vi "Connect.vi"(11 "Device Serial Number":string) -> (1 "Handle":u64, 3 "FT_Status":u64(ring) items=["FT_OK", "FT_INVALID_HANDLE", "FT_DEVICE_NOT_FOUND", "FT_DEVICE_NOT_OPENED", "FT_IO_ERROR", "FT_INSUFFICIENT_RESOURCES", "FT_INVALID_PARAMETER", "FT_INVALID_BAUD_RATE", "FT_DEVICE_NOT_OPENED_FOR_ERASE", "FT_DEVICE_NOT_OPENED_FOR_WRITE", "FT_FAILED_TO_WRITE_DEVICE", "FT_EEPROM_READ_FAILED", "FT_EEPROM_WRITE_FAILED", "FT_EEPROM_ERASE_FAILED", "FT_EEPROM_NOT_PRESENT", "FT_EEPROM_NOT_PROGRAMMED", "FT_INVALID_ARGS", "FT_NOT_SUPPORTED", "FT_OTHER_ERROR"])   [LabVIEW 2018]
panel:
  in  "Index":i64
  out "Count 3":i64
  out "Count 2":i64
  out "Count 1":i64
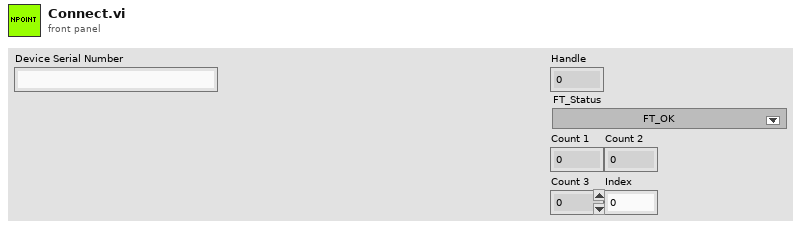
[diagram p1: front panel]
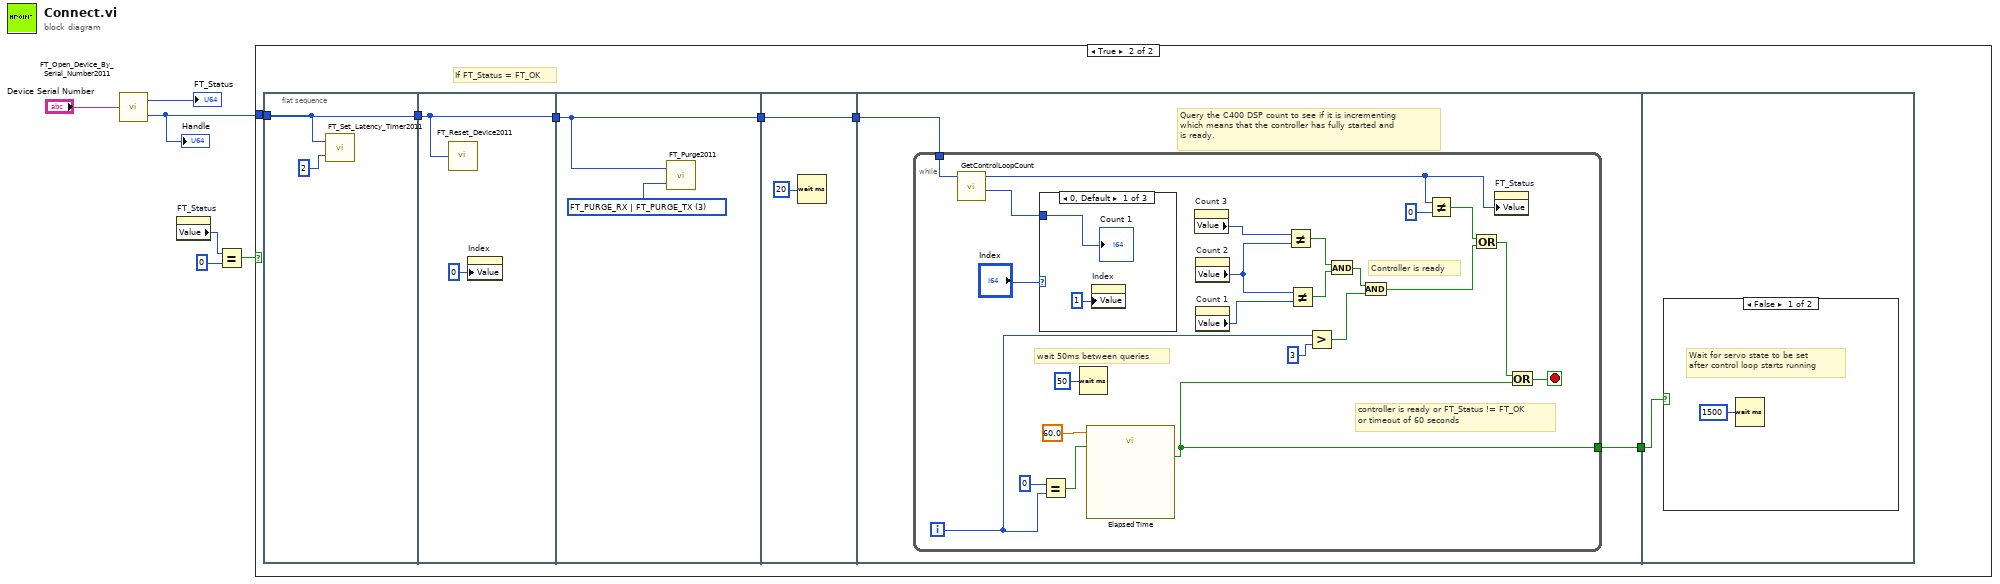
[diagram p0: block diagram]
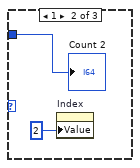
[diagram p3: hidden frame]
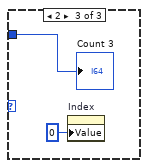
[diagram p4: hidden frame]
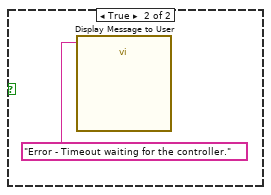
[diagram p5: hidden frame]
diagram:
  n1 = call "FT_Open_Device_By_Serial_Number2011.vi"("Device Serial Number"="Device Serial Number") -> ("FT_Status"=→"FT_Status":u64, "Handle"=w6:u64)
  "Handle" <- w6
  n2 = property on="FT_Status" class="Ring (strict)"() -> ("Value"=w2:u64)  [unwired: 2 in, 2 out]
  n3 = Equal?(x=w2, y=u64 0) -> (x = y?=w3:bool)
  n4 = case shown="True" w3 {
    tunnel: w6 -> [_ w12]
    frame False {
    }
    frame True {
      # "If FT_Status = FT_OK"
      n5 = flat-sequence {
        tunnel: w12 -> [w14]
        tunnel: [w14] -> w7
        tunnel: [w16] -> w11
        tunnel: w7 -> [w16]
        tunnel: w11 -> [w17]
        tunnel: [w17] -> w9
        tunnel: [w19] -> w10
        tunnel: w9 -> [w19]
        tunnel: w10 -> [w22]
        tunnel: [w21] -> w8
        tunnel: w8 -> [w52]
        frame #0 {
          n6 = call "FT_Set_Latency_Timer2011.vi"("Latency Timer Value"=u8 2, "Handle"=w14) -> ()  [unwired: 1 out]
        }
        frame #1 {
          n7 = call "FT_Reset_Device2011.vi"("Handle"=w16) -> ()  [unwired: 1 out]
          n8 = property on="Index" class="DigNum (strict)"("Value"=i64 0 ("Index")) -> ()  [unwired: 2 in, 2 out]
        }
        frame #2 {
          w18 = u64 3 items=["FT_PURGE_RX"=1, "FT_PURGE_TX"=2, "FT_PURGE_RX | FT_PURGE_TX"=3] ("Purge Flags")
          n9 = call "FT_Purge2011.vi"("Purge Flags"=w18, "Handle"=w17) -> ()  [unwired: 1 out]
        }
        frame #3 {
          n10 = Wait (ms)(milliseconds to wait=u32 20) -> ()  [unwired: 1 out]
        }
        frame #4 {
          # "Query the C400 DSP count to see if it is incrementing\nwhich means that the controller has fully started and \nis ready."
          n11 = while {
            tunnel: w22 -> [w45]
            tunnel: [w23] -> w21
            i -> [w26]
            stop <- w24 stop-if-true
            # "wait 50ms between queries"
            # "controller is ready or FT_Status != FT_OK\nor timeout of 60 seconds"
            # "Controller is ready"
            n12 = call "GetControlLoopCount.vi"("Handle"=w45) -> ("FT_Status"=w30:u64, "Control Loop Count"=w42:i64)  [unwired: 8 in]
            n13 = case shown="0, Default" "Index" {
              tunnel: w42 -> [w47 w49 w51]
              frame 0, Default {
                n14 = property on="Index" class="DigNum (strict)"("Value"=i64 1 ("Index")) -> ()  [unwired: 2 in, 2 out]
                "Count 1" <- w47
              }
              frame 1 {
                n15 = property on="Index" class="DigNum (strict)"("Value"=2 ("Index")) -> ()  [unwired: 2 in, 2 out]
                "Count 2" <- w49
              }
              frame 2 {
                n16 = property on="Index" class="DigNum (strict)"("Value"=0 ("Index")) -> ()  [unwired: 2 in, 2 out]
                "Count 3" <- w51
              }
            }
            n17 = Equal?(x=0, y=w26) -> (x = y?=w28:bool)
            n18 = Wait (ms)(milliseconds to wait=u32 50) -> ()  [unwired: 1 out]
            n19 = call "Elapsed Time"("Time Target (s)"=60.0, "Reset"=w28) -> ("Time has Elapsed"=w23:bool)  [unwired: 10 in, 7 out]
            n20 = property on="Count 3" class="DigNum (strict)"() -> ("Value"=w40:i64)  [unwired: 2 in, 2 out]
            n21 = property on="Count 2" class="DigNum (strict)"() -> ("Value"=w38:i64)  [unwired: 2 in, 2 out]
            n22 = property on="Count 1" class="DigNum (strict)"() -> ("Value"=w39:i64)  [unwired: 2 in, 2 out]
            n23 = Not Equal?(x=w40, y=w38) -> (x != y?=w37:bool)
            n24 = Not Equal?(x=w38, y=w39) -> (x != y?=w36:bool)
            n25 = Greater?(x=w26, y=3) -> (0:w35:bool)
            n26 = And(x=w37, y=w36) -> (x .and. y?=w34:bool)
            n27 = And(x=w34, y=w35) -> (x .and. y?=w32:bool)
            n28 = Not Equal?(x=w30, y=u64 0) -> (x != y?=w31:bool)
            n29 = Or(x=w31, y=w32) -> (x .or. y?=w25:bool)
            n30 = property on="FT_Status" class="Ring (strict)"("Value"=w30) -> ()  [unwired: 2 in, 2 out]
            n31 = Or(x=w25, y=w23) -> (x .or. y?=w24:bool)
          }
        }
        frame #5 {
          n32 = case shown="False" w52 {
            frame False {
              # "Wait for servo state to be set\nafter control loop starts running"
              n33 = Wait (ms)(milliseconds to wait=u32 1500) -> ()  [unwired: 1 out]
            }
            frame True {
              n34 = call "Display Message to User"("Message"="Error - Timeout waiting for the controller.") -> ()  [unwired: 9 in, 2 out]
            }
          }
        }
      }
    }
  }
